vi "Pump Info.vi"(7 "Pump ID (0:A)":T4, 8 "error in (no error)":errorcluster, 11 "VISA resource in":refnum<visa-resource-name>) -> (0 "error out":errorcluster, 1 "HW Flow Limits":T3, 2 "Session Info":T2, 3 "VISA resource out":refnum<visa-resource-name>)   [LabVIEW 2020, in "Global FIA milliGAT.lvlib"]
uses:
  <instrlib>/RxnRover/Global FIA milliGAT 3.14/Global FIA milliGAT.lvlib
  <instrlib>/RxnRover/Global FIA milliGAT 3.14/Public/Utility/Pump Address.ctl
  <instrlib>/RxnRover/Global FIA milliGAT 3.14/Public/Utility/Pump Direction.ctl
  <instrlib>/RxnRover/Global FIA milliGAT 3.14/Private/Pump Parameter.ctl
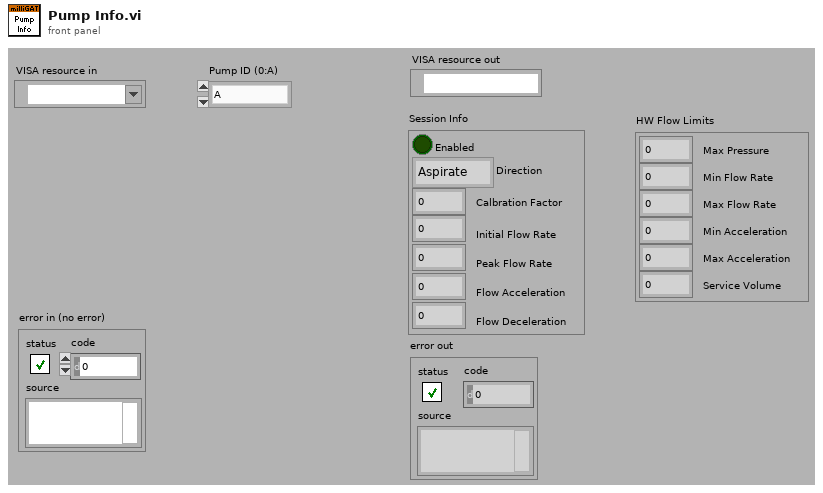
[diagram p1: front panel]
types:
  T1 = typedef "Global FIA milliGAT.lvlib/Pump Direction.ctl" = enum16{"Aspirate", "Dispense"}
  T2 = cluster{"Enabled":bool, "Direction":T1, "Calbration Factor":dbl, "Initial Flow Rate":dbl, "Peak Flow Rate":dbl, "Flow Acceleration":dbl, "Flow Deceleration":dbl}
  T3 = cluster{"Max Pressure":dbl, "Min Flow Rate":dbl, "Max Flow Rate":dbl, "Min Acceleration":dbl, "Max Acceleration":dbl, "Service Volume":dbl}
  T4 = typedef "Global FIA milliGAT.lvlib/Pump Address.ctl" = enum16{"A", "B", "C", "D", "E", "F", "G", "H", "I", "J", "K", "L", "M", "N", "O", "P", "Q", "R", "S", "T", "U", "V", "W", "X", "Y", "Z", "a", "b", "c", "d", "e", "f", "g", "h", "i", "j", "k", "l", "m", "n", "o", "p", "q", "r", "s", "t", "u", "v", "w", "x", "y", "z", "0", "1", "2", "3", "4", "5", "6", "7", "8", "9"}
  T5 = cluster{"Max Pressure":dbl, "Min Flow":dbl, "Max Flow":dbl, "Min Acceleration":dbl, "Max Acceleration":dbl, "Service Volume":dbl}
  T6 = typedef "Global FIA milliGAT.lvlib/Pump Parameter.ctl" = enum16{"Enabled", "EU", "EU Calibration Factor", "Fixed Asp or Disp", "Starting Position", "Starting Flow", "Peak Flow", "Flow Acceleration", "Flow Deceleration", "Session Volume", "Max Pressure", "Backlash (usteps)", "BL Calibration Factor", "BL Correction Enabled", "Min Flow", "Max Flow", "Min Acceleration", "Max Acceleration", "Service Volume", "Life Volume"}
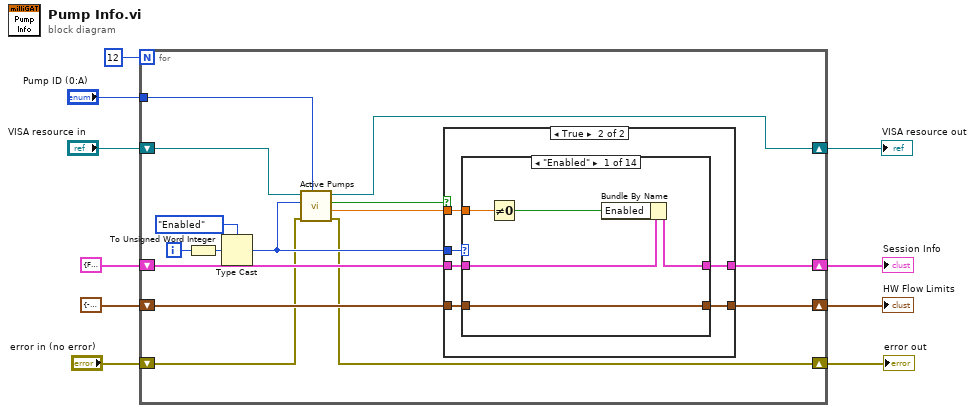
[diagram p0: block diagram]
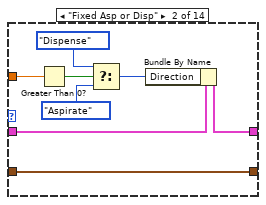
[diagram p3: hidden frame]
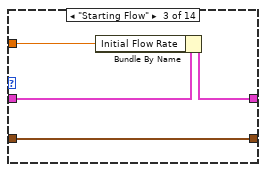
[diagram p4: hidden frame]
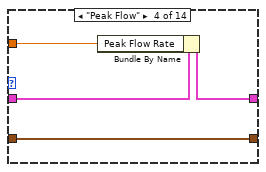
[diagram p5: hidden frame]
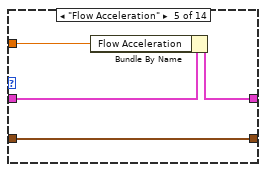
[diagram p6: hidden frame]
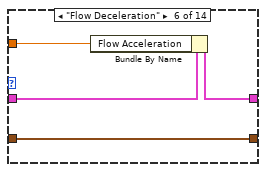
[diagram p7: hidden frame]
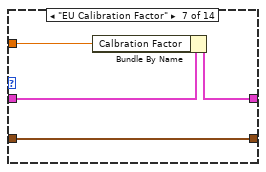
[diagram p8: hidden frame]
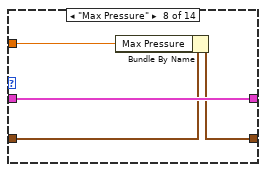
[diagram p9: hidden frame]
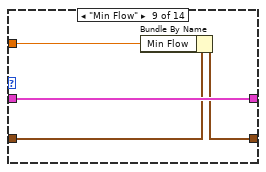
[diagram p10: hidden frame]
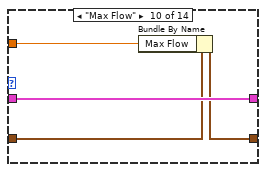
[diagram p11: hidden frame]
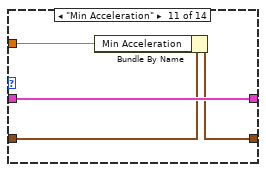
[diagram p12: hidden frame]
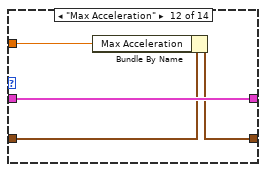
[diagram p13: hidden frame]
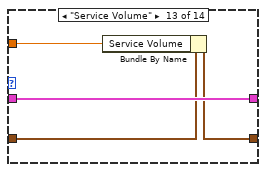
[diagram p14: hidden frame]
diagram:
  n1 = for {
    N: 12 -> [_]
    shift-right: [w20] -> w6
    shift-left: T2 {"Enabled"=FALSE, "Direction"=enum."Dispense", "Calbration Factor"=0.0, "Initial Flow Rate"=0.0, "Peak Flow Rate"=0.0, "Flow Acceleration"=0.0, "Flow Deceleration"=0.0} ("Session Info") -> [w21]
    shift-right: [w19] -> w8
    shift-left: T5 {"Max Pressure"=-1.0, "Min Flow"=-1.0, "Max Flow"=-1.0, "Min Acceleration"=-1.0, "Max Acceleration"=-1.0, "Service Volume"=-1.0} ("Flow Configuration") -> [w18]
    tunnel: "Pump ID (0:A)" -> [w22]
    shift-right: [w13] -> w3
    shift-left: "VISA resource in" -> [w14]
    shift-right: [w11] -> w1
    shift-left: "error in (no error)" -> [w12]
    i -> [w25]
    n2 = To Unsigned Word Integer(number=w25) -> (unsigned 16bit integer=w15:u16)
    n3 = Type Cast(type=Pump_Parameter."Enabled" ("Parameter (0:Enabled)"), x=w15) -> (*(type *) &x=w23:T6)
    n4 = call <instrlib>:"Active Pumps.vi"("Pump ID (0:A)"=w22, "error in (no error)"=w12, "Parameter"=w23, "VISA resource in"=w14) -> ("error out"=w11:errorcluster, "Value out"=w17:dbl, "Found"=w16:bool, "VISA resource out"=w13:refnum<visa-resource-name>)  [unwired: 4 in]
    n5 = case shown="True" w16 {
      tunnel: w23 -> [_ w33]
      tunnel: w21 -> [w27 w32]
      tunnel: [w27 w31] -> w20
      tunnel: [w26 w30] -> w19
      tunnel: w18 -> [w26 w29]
      tunnel: w17 -> [_ w28]
      frame False {
        # "Not Found"
      }
      frame True {
        n6 = case shown="\"Enabled\"" w33 {
          tunnel: w32 -> [w36 w44 w48 w52 w56 w60 w64 w69 w73 w77 w81 w85 w89 w92]
          tunnel: [w37 w45 w49 w53 w57 w61 w65 w69 w73 w77 w81 w85 w89 w92] -> w31
          tunnel: [w38 w46 w50 w54 w58 w62 w66 w67 w71 w75 w79 w83 w87 w91] -> w30
          tunnel: w29 -> [w38 w46 w50 w54 w58 w62 w66 w68 w72 w76 w80 w84 w88 w91]
          tunnel: w28 -> [w35 w43 w47 w51 w55 w59 w63 w70 w74 w78 w82 w86 w90 _]
          frame "Enabled" {
            n7 = Not Equal To 0?(x=w35) -> (x != 0?=w34:bool)
            n8 = Bundle By Name(cluster=w36, "Enabled"=w34) -> (w37:T2)
          }
          frame "Fixed Asp or Disp" {
            n9 = Greater Than 0?(x=w43) -> (x > 0?=w42:bool)
            n10 = Select(t=Pump_Direction."Dispense" ("Direction"), s=w42, f=Pump_Direction."Aspirate" ("Direction")) -> (s? t:f=w41:T1)
            n11 = Bundle By Name(cluster=w44, "Direction"=w41) -> (w45:T2)
          }
          frame "Starting Flow" {
            n12 = Bundle By Name(cluster=w48, "Initial Flow Rate"=w47) -> (w49:T2)
          }
          frame "Peak Flow" {
            n13 = Bundle By Name(cluster=w52, "Peak Flow Rate"=w51) -> (w53:T2)
          }
          frame "Flow Acceleration" {
            n14 = Bundle By Name(cluster=w56, "Flow Acceleration"=w55) -> (w57:T2)
          }
          frame "Flow Deceleration" {
            n15 = Bundle By Name(cluster=w60, "Flow Acceleration"=w59) -> (w61:T2)
          }
          frame "EU Calibration Factor" {
            n16 = Bundle By Name(cluster=w64, "Calbration Factor"=w63) -> (w65:T2)
          }
          frame "Max Pressure" {
            n17 = Bundle By Name(cluster=w68, "Max Pressure"=w70) -> (w67:T5)
          }
          frame "Min Flow" {
            n18 = Bundle By Name(cluster=w72, "Min Flow"=w74) -> (w71:T5)
          }
          frame "Max Flow" {
            n19 = Bundle By Name(cluster=w76, "Max Flow"=w78) -> (w75:T5)
          }
          frame "Min Acceleration" {
            n20 = Bundle By Name(cluster=w80, "Min Acceleration"=w82) -> (w79:T5)
          }
          frame "Max Acceleration" {
            n21 = Bundle By Name(cluster=w84, "Max Acceleration"=w86) -> (w83:T5)
          }
          frame "Service Volume" {
            n22 = Bundle By Name(cluster=w88, "Service Volume"=w90) -> (w87:T5)
          }
          frame Default {
          }
        }
      }
    }
  }
  "HW Flow Limits" <- w8
  "Session Info" <- w6
  "VISA resource out" <- w3
  "error out" <- w1
